vi "FrameworkHL.vi"(7 "StandardRequests":refnum<event-registration>, 10 "Message Queue":refnum<class "RQMHMessageQueue.lvclass">, 11 "JQMHModule in":refnum<class "RQMHModule.lvclass">) -> ()   [LabVIEW 2024, in "RQMHModule.lvclass"]
doc: "Helper loop for framework tasks"
uses:
  RQMHModule.lvclass
  Message Queue_class/RQMHMessageQueue.lvclass
  StandardRequests.ctl
  InitialiseArgs.ctl
  Reply.ctl
  StopEventArgs.ctl
  Show Front Panel--Args.ctl
  Hide Front Panel.ctl
  Show Block Diagram.ctl
  Hide Block Diagram--Args.ctl
  Message Queue_class/RQMHMessageQueue.lvclass/RQMHMessageQueue.ctl
  RQMHModule.lvclass/RQMHModule.ctl
  Message Queue_class/Delacor_lib_QMH_Enqueue Message (Single).vi
  Shared/JQMHShared.lvlib
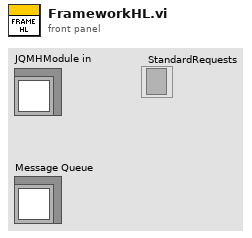
[diagram p1: front panel]
types:
  T1 = enum32{"Invalid", "Standard", "Closed", "Hidden", "Minimized", "Maximized"}
  T2 = typedef "RQMHModule.lvclass/InitialiseArgs.ctl" = cluster{"null":bool}
  T3 = typedef "RQMHModule.lvclass/Reply.ctl" = cluster{"Expects Reply":bool, "Reply":refnum<notifier>}
  T4 = typedef "RQMHModule.lvclass/Show Front Panel--Args.ctl" = variant
  T5 = typedef "RQMHModule.lvclass/Show Block Diagram.ctl" = bool
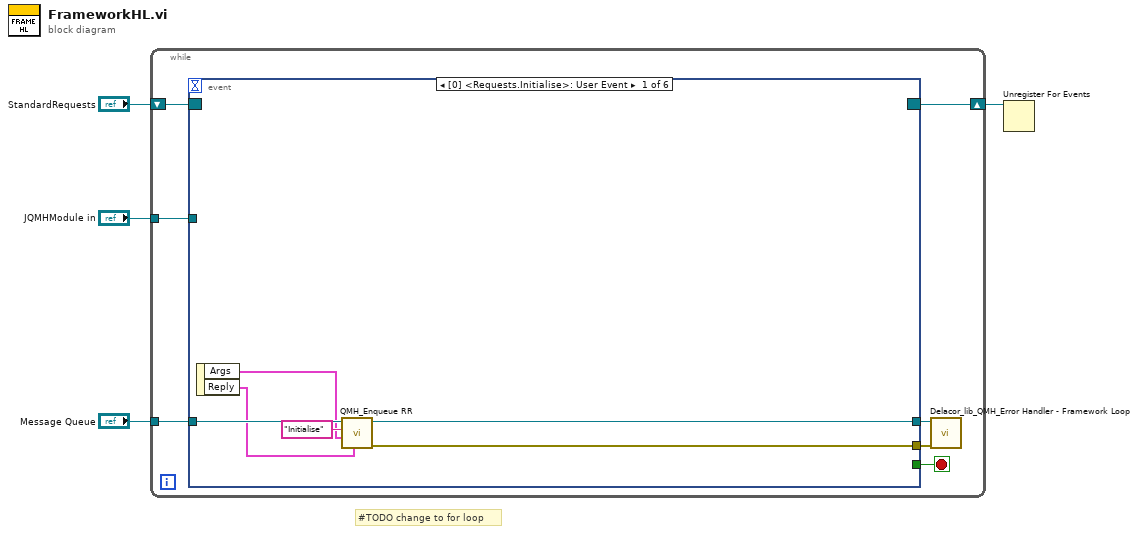
[diagram p0: block diagram]
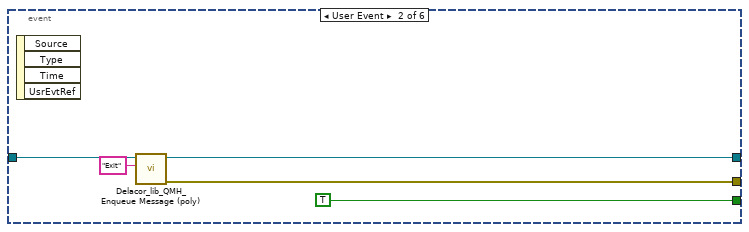
[diagram p2: hidden frame]
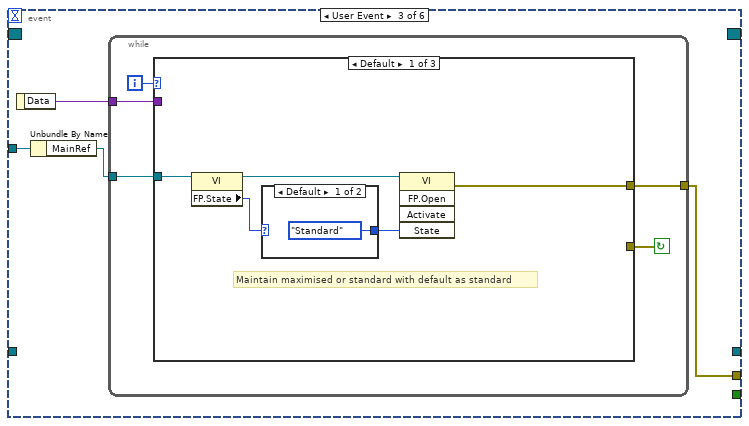
[diagram p3: hidden frame]
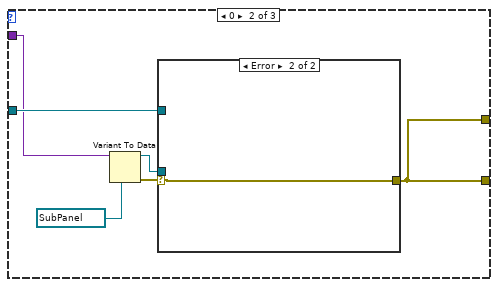
[diagram p5: hidden frame]
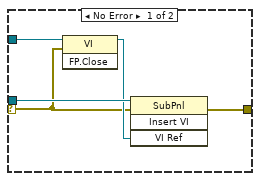
[diagram p6: hidden frame]
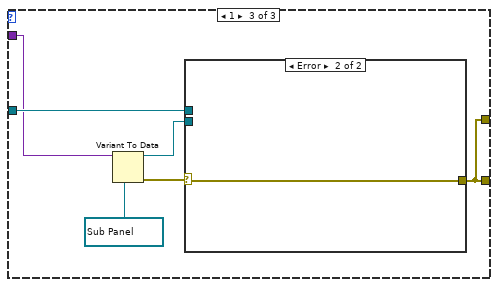
[diagram p7: hidden frame]
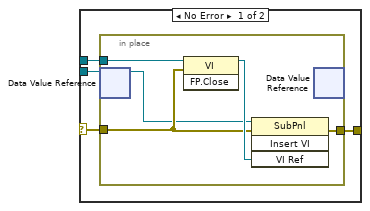
[diagram p8: hidden frame]
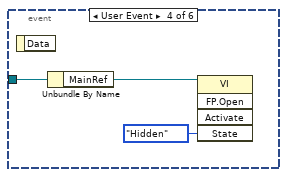
[diagram p9: hidden frame]
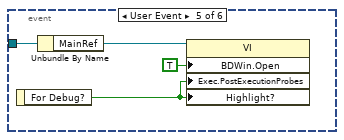
[diagram p10: hidden frame]
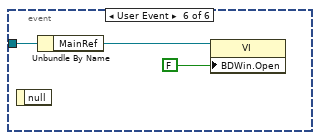
[diagram p11: hidden frame]
diagram:
  # "#TODO change to for loop"
  n1 = while {
    shift-right: [w11] -> w4
    shift-left: "StandardRequests" -> [w5]
    tunnel: "Message Queue" -> [w10]
    tunnel: "JQMHModule in" -> [w6]
    stop <- w7 stop-if-true
    n2 = event shown="[0] <Requests.Initialise>: User Event" {
      selector: w5 -> [_ _ _ _ _ _]
      dyn-events: [_ _ _ _ _ _] -> w11
      timeout: _ -> [_ _ _ _ _ _]
      tunnel: w10 -> [w17 w20 _ _ _ _]
      tunnel: [w16 w19 _ _ _ _] -> w9
      tunnel: [w15 w18 w23 _ _ _] -> w8
      tunnel: [_ TRUE _ _ _ _] -> w7
      tunnel: w6 -> [_ _ w26 w69 w73 w76]
      event User Event {
        n3 = event-data() -> ("Args"=w13:T2, "Reply"=w12:T3)  [unwired: 1 in]
        n4 = call "QMH_Enqueue RR.vi"("Reply"=w12, "Message Data"=w13, "Message"="Initialise", "Message Queue in"=w17) -> ("error out"=w15:errorcluster, "Message Queue out"=w16:refnum<class "RQMHMessageQueue.lvclass">)  [unwired: 6 in]
      }
      event User Event {
        n5 = event-data() -> ()  [unwired: 1 in, 4 out]
        n6 = call-poly "Delacor_lib_QMH_Enqueue Message (poly).vi"("Message"="Exit", "Message Queue in"=w20) -> ("error out"=w18:errorcluster, "Message Queue out"=w19:refnum<class "RQMHMessageQueue.lvclass">)  [unwired: 8 in]
      }
      event User Event {
        n7 = event-data() -> ("Data"=w24:T4)  [unwired: 1 in]
        n8 = Unbundle By Name(w26) -> ("MainRef"=w25:refnum<vi>)
        n9 = while {
          tunnel: w25 -> [w30]
          tunnel: [w28] -> w23
          tunnel: w24 -> [w27]
          i -> [w31]
          stop <- w29 continue-if-true
          n10 = case shown="Default" w31 {
            tunnel: w30 -> [w36 w44 w56]
            tunnel: [_ w43 w55] -> w29
            tunnel: w27 -> [_ w40 w54]
            tunnel: [w35 w43 w55] -> w28
            frame Default {
              # "Maintain maximised or standard with default as standard"
              n11 = property class="VI"(reference=w36) -> (reference out=w34:refnum<vi>, "FP.State"=w33:T1)  [unwired: 1 in, 1 out]
              n12 = case shown="Default" w33 {
                selector: w33 -> [_ w38]
                tunnel: [T1."Standard" ("FP.State") w38] -> w32
                frame Default {
                }
                frame "Standard", "Maximized" {
                }
              }
              n13 = invoke class="VI" method="FP.Open"(reference=w34, "State"=w32) -> (error out=w35:errorcluster)  [unwired: 3 in, 4 out]
            }
            frame 0 {
              n14 = Variant To Data(type=refnum<vi> refnum ("Sub Panel"), Variant=w40) -> (data=w41:refnum<vi>, error out=w42:errorcluster)  [unwired: 1 in]
              n15 = case shown="Error" w42 {
                selector: w42 -> [w45 w50]
                tunnel: w41 -> [w49 _]
                tunnel: w44 -> [w48 _]
                tunnel: [w46 w50] -> w43
                frame No Error {
                  n16 = invoke class="VI" method="FP.Close"(reference=w48, error in=w45) -> (reference out=w47:refnum<vi>)  [unwired: 1 in, 2 out]
                  n17 = invoke class="SubPnl" method="Insert VI"(reference=w49, error in=w45, "VI Ref"=w47) -> (error out=w46:errorcluster)  [unwired: 1 in, 3 out]
                }
                frame Error {
                }
              }
            }
            frame 1 {
              n18 = Variant To Data(type=refnum<data-value> refnum ("data value reference"), Variant=w54) -> (data=w51:refnum<data-value>, error out=w52:errorcluster)  [unwired: 1 in]
              n19 = case shown="Error" w52 {
                selector: w52 -> [w58 w66]
                tunnel: w56 -> [w60 _]
                tunnel: [w59 w66] -> w55
                tunnel: w51 -> [w57 _]
                frame No Error {
                  n20 = in-place {
                    in-place-border: w60 -> [w65]
                    in-place-border: [w63] -> w59
                    in-place-border: w58 -> [w62]
                    n21 = in-place-dvr #1(w57) -> (w61:refnum<vi>)  [unwired: 1 out]
                    n22 = invoke class="VI" method="FP.Close"(reference=w65, error in=w62) -> (reference out=w64:refnum<vi>)  [unwired: 1 in, 2 out]
                    n23 = invoke class="SubPnl" method="Insert VI"(reference=w61, error in=w62, "VI Ref"=w64) -> (error out=w63:errorcluster)  [unwired: 1 in, 3 out]
                    n24 = in-place-dvr #1() -> ()  [unwired: 1 in, 2 out]
                  }
                }
                frame Error {
                }
              }
            }
          }
        }
      }
      event User Event {
        n25 = event-data() -> ()  [unwired: 1 in, 1 out]
        n26 = Unbundle By Name(w69) -> ("MainRef"=w68:refnum<vi>)
        n27 = invoke class="VI" method="FP.Open"(reference=w68, "State"=T1."Hidden") -> ()  [unwired: 3 in, 5 out]
      }
      event User Event {
        n28 = event-data() -> ("For Debug?"=w71:T5)  [unwired: 1 in]
        n29 = Unbundle By Name(w73) -> ("MainRef"=w72:refnum<vi>)
        n30 = property class="VI"(reference=w72, "BDWin.Open"=TRUE ("Block Diagram Window:Open"), "Exec.PostExecutionProbes"=w71, "Highlight?"=w71) -> ()  [unwired: 1 in, 2 out]
      }
      event User Event {
        n31 = event-data() -> ()  [unwired: 1 in, 1 out]
        n32 = Unbundle By Name(w76) -> ("MainRef"=w75:refnum<vi>)
        n33 = property class="VI"(reference=w75, "BDWin.Open"=FALSE ("Block Diagram Window:Open")) -> ()  [unwired: 1 in, 2 out]
      }
    }
    n34 = call-dynamic "Delacor_lib_QMH_Error Handler - Framework Loop.vi"("error in"=w8, "Message Queue in"=w9) -> ()  [unwired: 8 in, 2 out]
  }
  n35 = Unregister For Events(event registration refnum=w4) -> ()  [unwired: 1 in, 1 out]
